vi "Timeout.vi"(8 "error in (no error)":errorcluster, 11 "LargeScrollbar in":refnum<class "LargeScrollbar.lvclass">) -> (0 "error out":errorcluster)   [LabVIEW 2015, in "LargeScrollbar.lvclass"]
doc: "<b> </b> <b> </b>\n©2016 Q Software Innovations, LLC (QSI)\nwritten by Quentin Alldredge\nproduced in LabVIEW 2015\n\nsupport@qsoftwareinnovations.com\nwww.qsoftwareinnovations.com\n\nAll rights reserved.\n\nRedistribution and use in source and binary forms, with or without modification, are permitted provided that the following conditions are met:\n\n * Redistributions of source code must retain the above copyright notice, this list of conditions and the following disclaimer.\n * Redistributions in binary form must reproduce the above copyright notice, this list of conditions and the following disclaimer in the documentation and/or other materials provided with the distribution.\n * Neither the name of Q Software Innovations, LLC. nor the names of its contributors may be used to endorse or promote products derived from this software without specific prior written permission.\n\nTHIS SOFTWARE IS PROVIDED BY THE COPYRIGHT HOLDERS AND CONTRIBUTORS \"AS IS\" AND ANY EXPRESS OR IMPLIED WARRANTIES, INCLUDING, BUT NOT LIMITED TO, THE IMPLIED WARRANTIES OF MERCHANTABILITY AND FITNESS FOR A PARTICULAR PURPOSE ARE DISCLAIMED. IN NO EVENT SHALL THE COPYRIGHT OWNER OR CONTRIBUTORS BE LIABLE FOR ANY DIRECT, INDIRECT, INCIDENTAL, SPECIAL, EXEMPLARY, OR CONSEQUENTIAL DAMAGES (INCLUDING, BUT NOT LIMITED TO, PROCUREMENT OF SUBSTITUTE GOODS OR SERVICES; LOSS OF USE, DATA, OR PROFITS; OR BUSINESS INTERRUPTION) HOWEVER CAUSED AND ON ANY THEORY OF LIABILITY, WHETHER IN CONTRACT, STRICT LIABILITY, OR TORT (INCLUDING NEGLIGENCE OR OTHERWISE) ARISING IN ANY WAY OUT OF THE USE OF THIS SOFTWARE, EVEN IF ADVISED OF THE POSSIBILITY OF SUCH DAMAGE."
uses:
  LargeScrollbar.lvclass
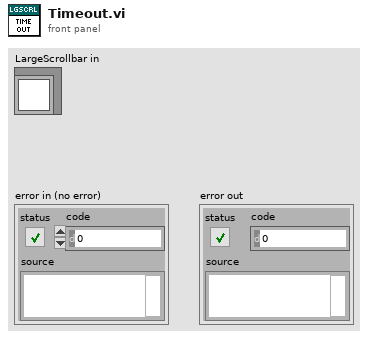
[diagram p1: front panel]
types:
  T1 = typedef "LargeScrollbar.lvclass/Direction.ctl" = enum16{"Decrement", "Increment"}
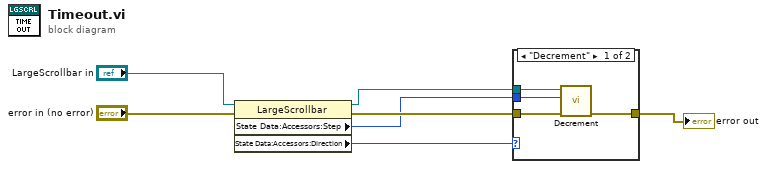
[diagram p0: block diagram]
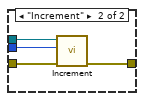
[diagram p2: hidden frame]
diagram:
  n1 = property class="LargeScrollbar"(reference="LargeScrollbar in", error in="error in (no error)") -> (reference out=w3:refnum<class "LargeScrollbar.lvclass">, error out=w5:errorcluster, "State Data:Accessors:Step"=w2:i32, "State Data:Accessors:Direction"=w1:T1)
  n2 = case shown="\"Decrement\"" w1 {
    tunnel: w3 -> [w11 w15]
    tunnel: w5 -> [w10 w14]
    tunnel: [w9 w13] -> w7
    tunnel: w2 -> [w8 w12]
    frame "Decrement" {
      n3 = call "Decrement.vi"("error in (no error)"=w10, "Step (1)"=w8, "LargeScrollbar in"=w11) -> ("error out"=w9:errorcluster)  [unwired: 8 in]
    }
    frame "Increment" {
      n4 = call "Increment.vi"("error in (no error)"=w14, "Step (1)"=w12, "LargeScrollbar in"=w15) -> ("error out"=w13:errorcluster)  [unwired: 8 in]
    }
  }
  "error out" <- w7
